vi "Write Default Service Settings File.vi"(8 "error in (no error)":errorcluster) -> (0 "error out":errorcluster, 3 "service settings":T1={"port"=56789, "enable debug log"=FALSE})   [LabVIEW 2021, in "AudioGenUtility.lvlib"]
uses:
  AudioGenUtility.lvlib
  controls/service settings.ctl
  controls/AudioGenTypeDefs.lvlib
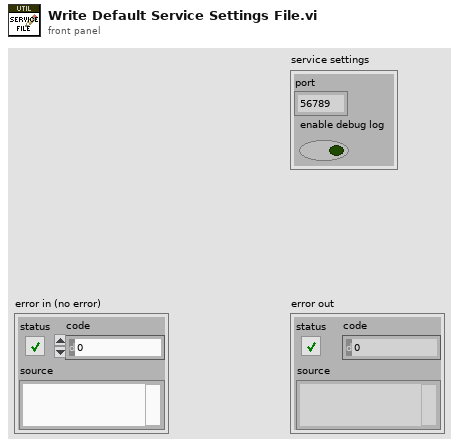
[diagram p1: front panel]
types:
  T1 = typedef "AudioGenTypeDefs.lvlib/service settings.ctl" = cluster{"port":u32, "enable debug log":bool}
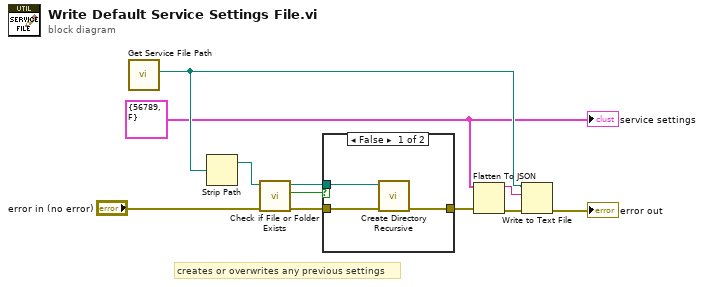
[diagram p0: block diagram]
diagram:
  w2 = T1 {"port"=56789, "enable debug log"=FALSE} ("service settings")
  # "creates or overwrites any previous settings"
  n1 = call "Get Service File Path.vi"() -> ("service setting file"=w4:path)  [unwired: 11 in]
  n2 = Strip Path(path=w4) -> (stripped path=w5:path)  [unwired: 1 out]
  n3 = call <vilib>:"Check if File or Folder Exists.vi"("error in (no error)"="error in (no error)", "path"=w5) -> ("error out"=w8:errorcluster, "file or folder exists?"=w9:bool, "dup path"=w1:path)  [unwired: 7 in]
  n4 = case shown="False" w9 {
    tunnel: w8 -> [w14 w15]
    tunnel: [w13 w15] -> w3
    tunnel: w1 -> [w12 _]
    frame False {
      n5 = call <vilib>:"Create Directory Recursive.vi"("error in (no error)"=w14, "directory"=w12) -> ("error out"=w13:errorcluster)  [unwired: 3 in, 2 out]
    }
    frame True {
    }
  }
  n6 = Flatten To JSON(anything=w2, error in (no error)=w3) -> (JSON string=w7:string, 11:w6:errorcluster)  [unwired: 1 in]
  n7 = Write to Text File(file (use dialog)=w4, text=w7, error in=w6) -> (error out=→"error out":errorcluster)  [unwired: 1 in, 2 out]
  "service settings" <- w2
